vi "Get Internal Byte Stream.vi"(8 "error in (no error)":errorcluster, 11 "Buffer Data in":refnum<class "Buffer.lvclass">) -> (0 "error out":errorcluster, 2 "Byte Stream":refnum<data-value>, 3 "Buffer Data":refnum<class "Buffer.lvclass">)   [LabVIEW 2020, in "Buffer.lvclass"]
doc: "This exposes the buffer's internal byte-stream for use with IMAQ's \"ByteStreamToImage\".\n\nDeleting this External DVR will cause the buffer to be destroyed so it is advised to not attempt to delete this EDVR. The internal resources will be cleaned up as necessary."
uses:
  Buffer.lvclass
  Buffer.lvclass/Buffer.ctl
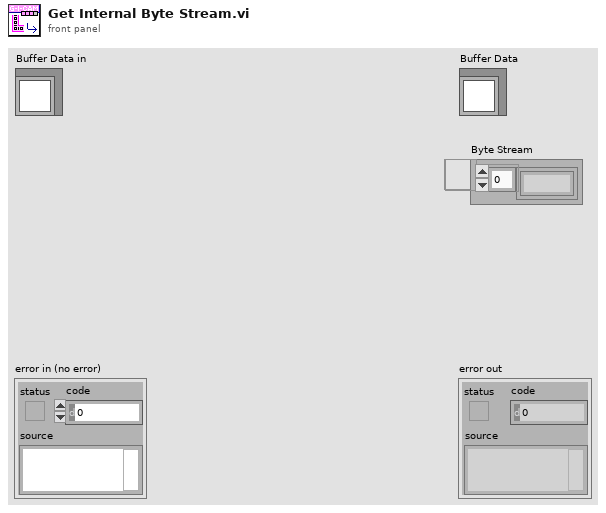
[diagram p1: front panel]
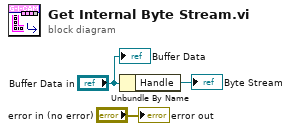
[diagram p0: block diagram]
diagram:
  n1 = Unbundle By Name("Buffer Data in") -> ("Handle"=→"Byte Stream":refnum<data-value>)
  "error out" <- "error in (no error)"
  "Buffer Data" <- "Buffer Data in"
